vi "Init AC Source.vi"(6 "General Settings:Timeout Value":u32=2000, 8 "error in (no error)":errorcluster, 9 "AC sync source":T1, 11 "AC source":T1) -> (0 "error out":errorcluster, 1 "AC sync source out":T1, 2 "Init status":string, 3 "AC source out":T1)   [LabVIEW 2020]
doc: "Initialize the driver of the selected AC source."
uses:
  Type definitions/AC Source.ctl
  Type definitions/AC Source type.ctl
  external libraries/Fluke 5XXX Series Multicalibrator/Fluke 5XXX Series Multicalibrators.lvlib
  external libraries/AWG/AFG3000/Tektronix AFG 3000 Series.lvlib
  external libraries/AWG/Agilent 33XXX Series/Agilent 33XXX Series.lvlib
  external libraries/AWG/Agilent 3352X Series/Agilent 3352X Series.lvlib
panel:
  in  "General Settings:Timeout Value 2":u32=2000
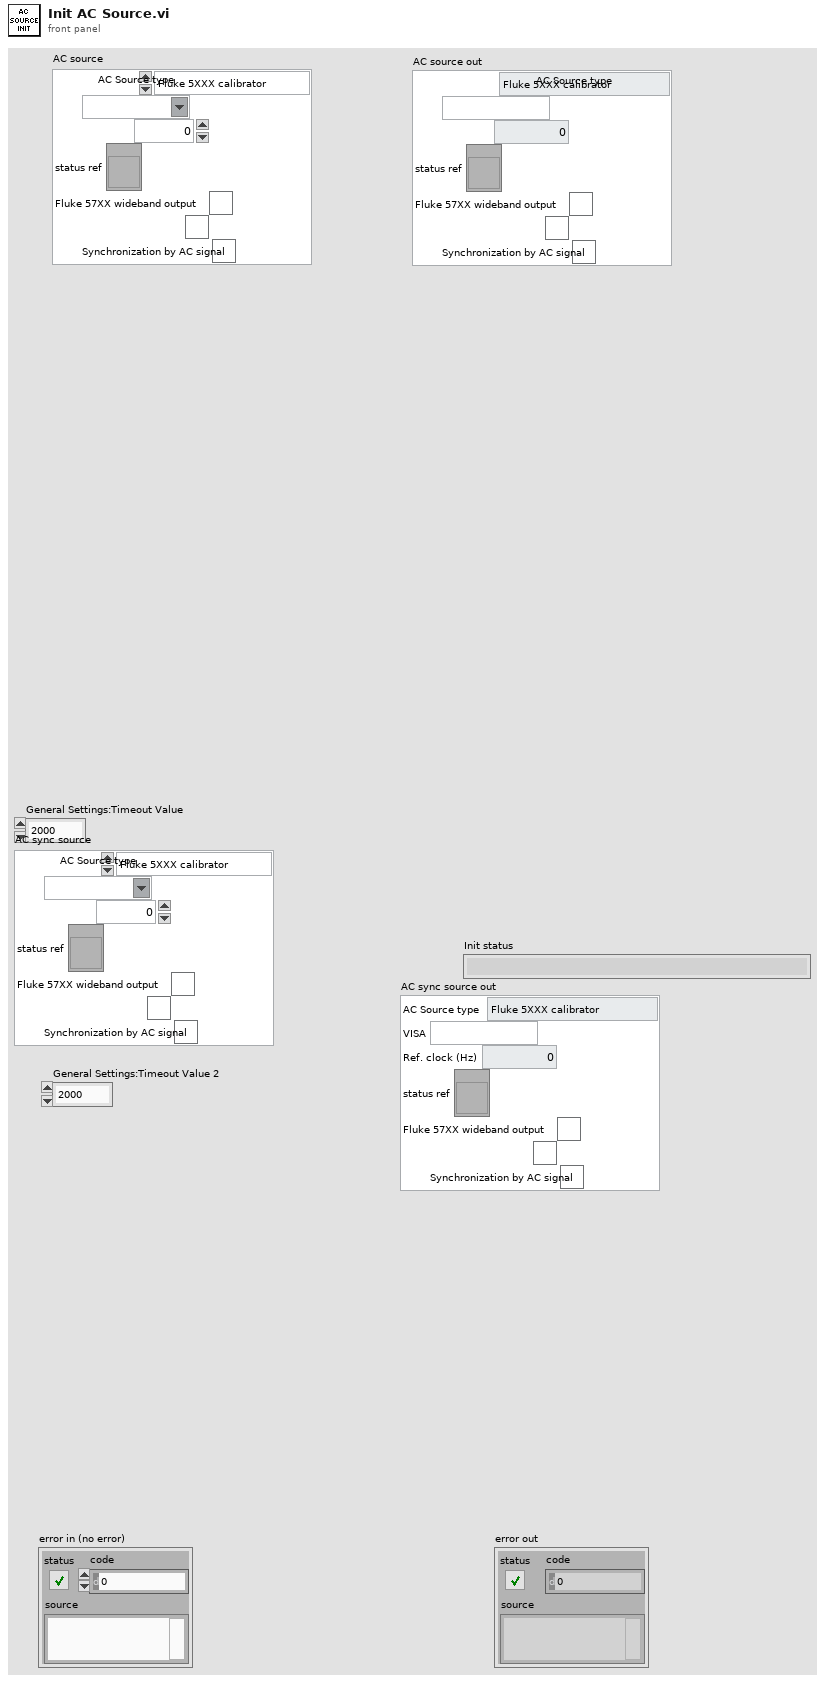
[diagram p1: front panel]
types:
  T1 = typedef "AC Source.ctl" = cluster{"AC Source type":T2, "VISA":refnum<visa-resource-name>, "Ref. clock (Hz)":dbl, "status ref":refnum<vi>, "Fluke 57XX wideband output":bool, "Fluke 57XX ignore errors":bool, "Synchronization by AC signal":bool}
  T2 = typedef "AC Source type.ctl" = enum16{"Fluke 5XXX calibrator", "Tektronix AFG3000 series", "dummy", "Agilent 331xxA to 332xxA", "Agilent 335xxA to 336xxA"}
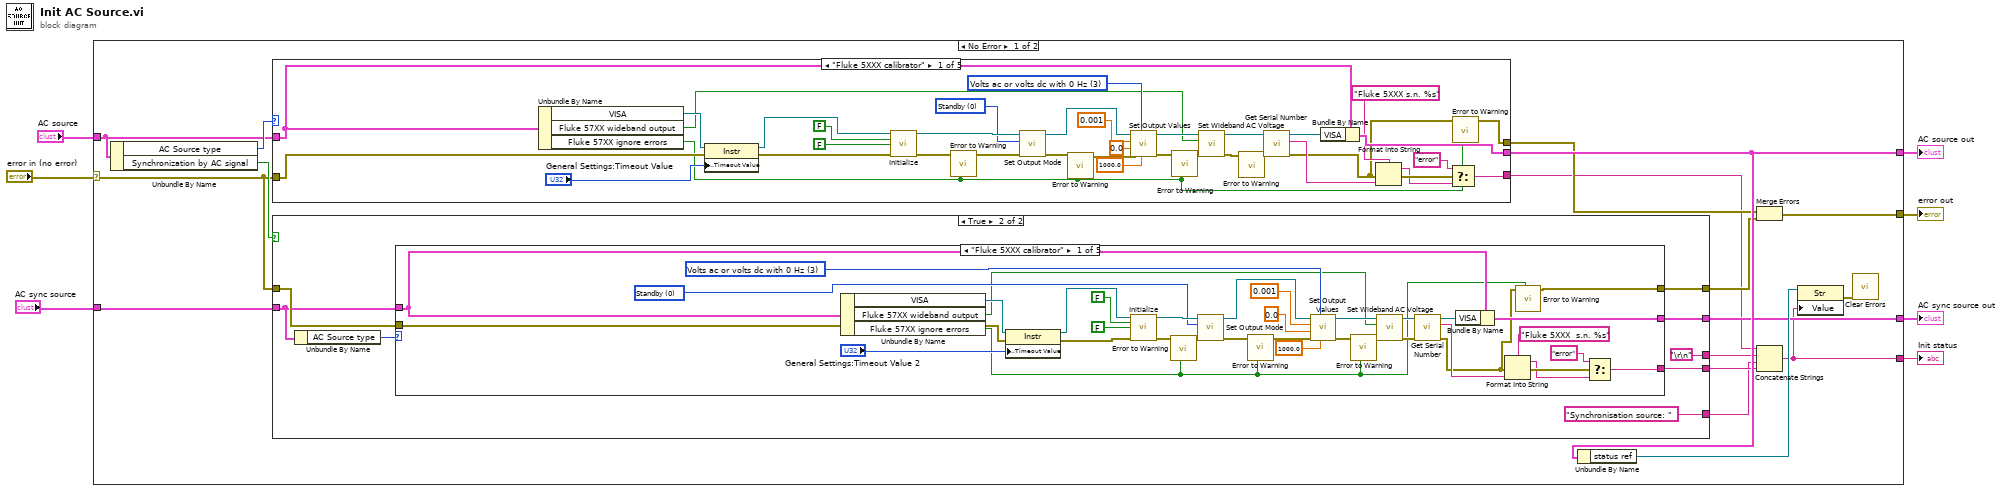
[diagram p0: block diagram]
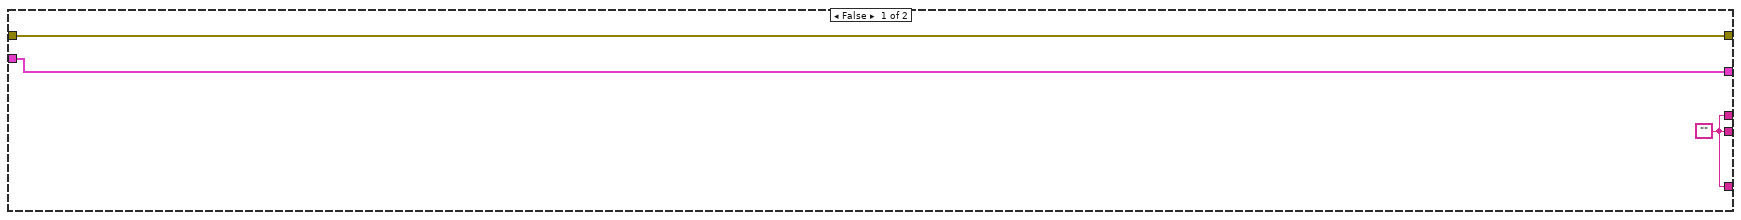
[diagram p2: hidden frame]
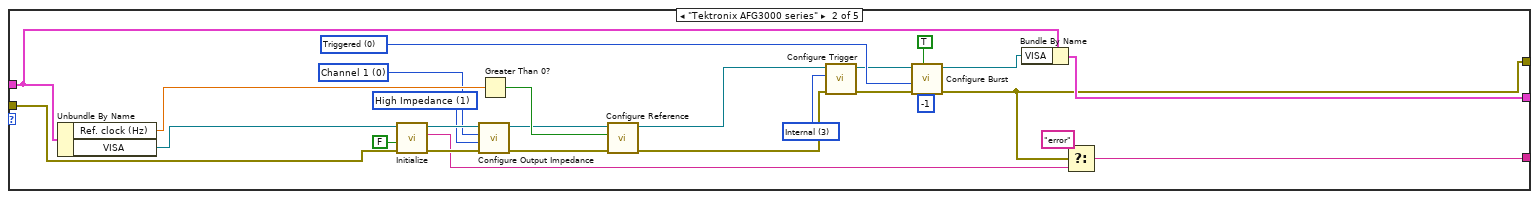
[diagram p3: hidden frame]
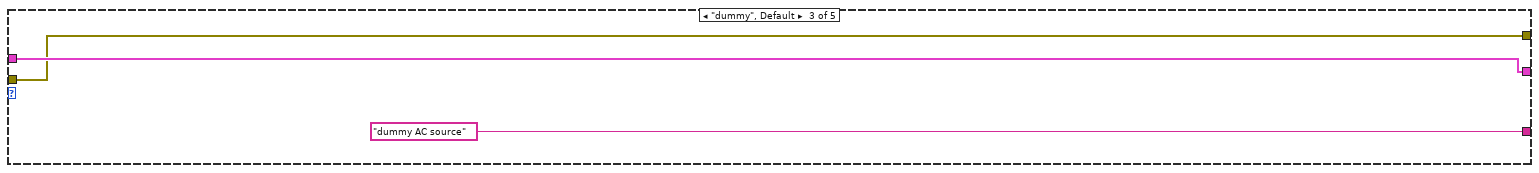
[diagram p4: hidden frame]
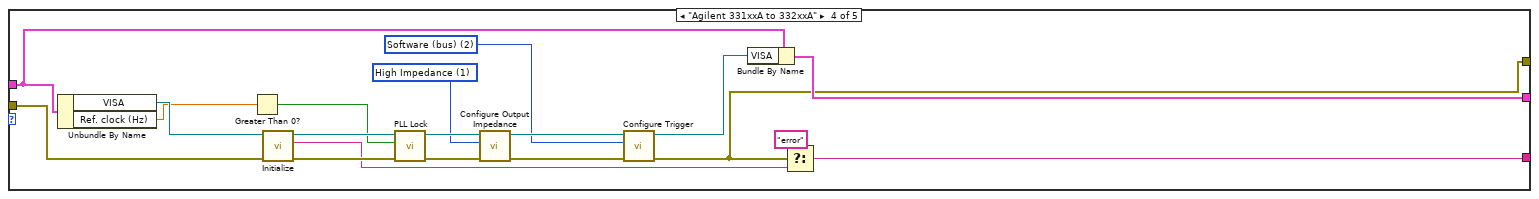
[diagram p5: hidden frame]
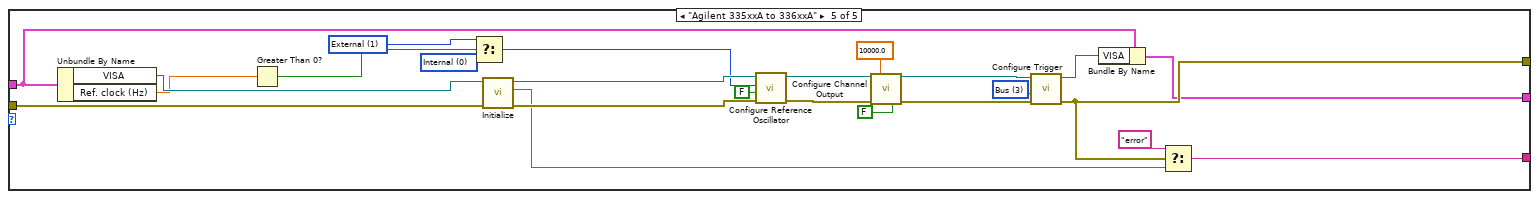
[diagram p6: hidden frame]
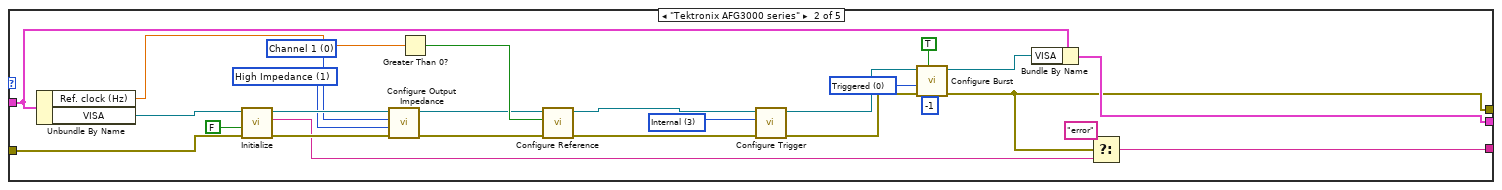
[diagram p7: hidden frame]
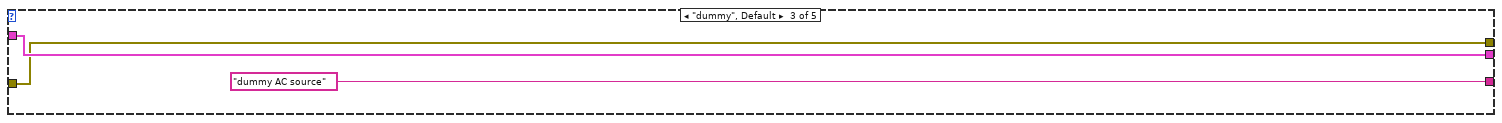
[diagram p8: hidden frame]
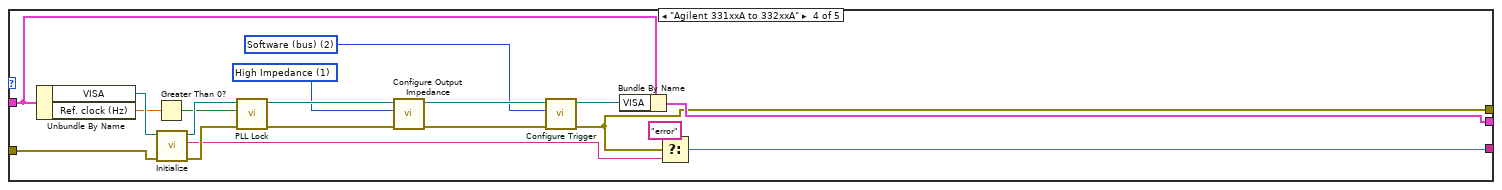
[diagram p9: hidden frame]
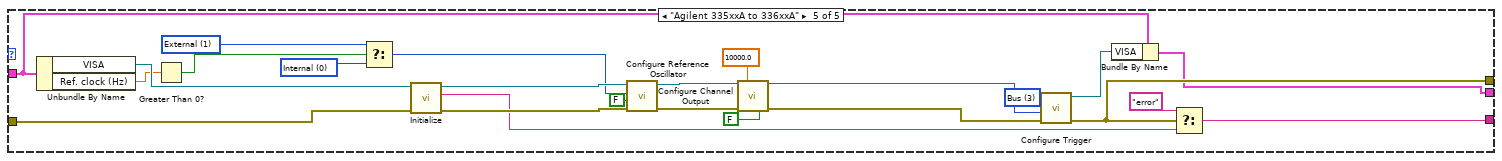
[diagram p10: hidden frame]
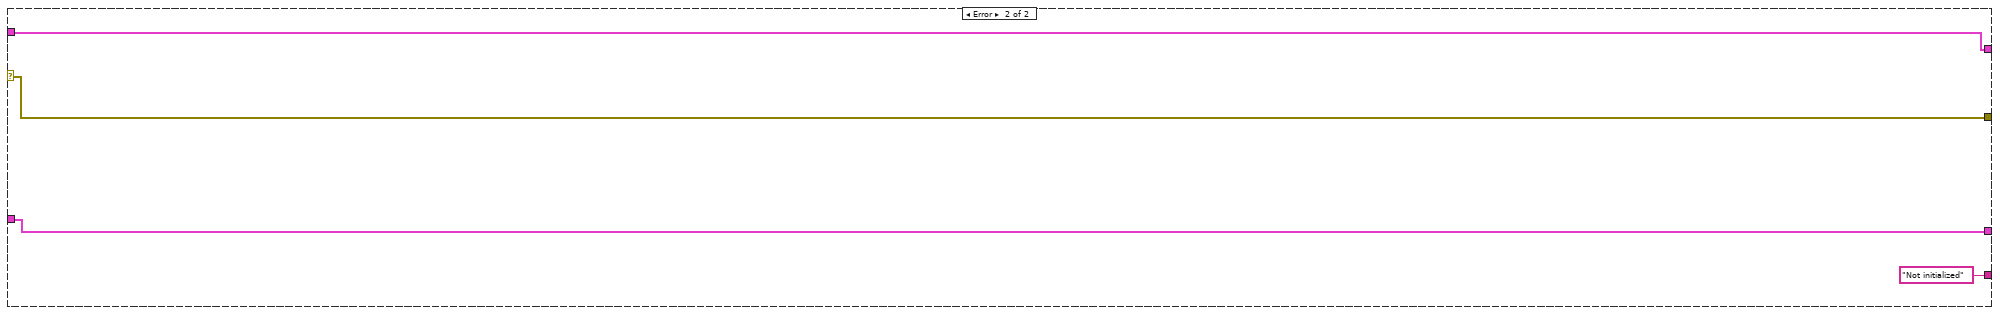
[diagram p11: hidden frame]
diagram:
  n1 = case shown="No Error" "error in (no error)" {
    selector: "error in (no error)" -> [w17 w255]
    tunnel: [w13 w255] -> w7
    tunnel: "AC source" -> [w23 w256]
    tunnel: [w22 w256] -> w5
    tunnel: [w11 "Not initialized" ("idn string")] -> w4
    tunnel: "AC sync source" -> [w18 w253]
    tunnel: [w16 w253] -> w1
    frame No Error {
      n2 = Unbundle By Name(w23) -> ("AC Source type"=w24:T2, "Synchronization by AC signal"=w19:bool)
      n3 = case shown="\"Fluke 5XXX calibrator\"" w24 {
        tunnel: w17 -> [w163 w200 w208 w220 w235]
        tunnel: [w145 w183 w208 w212 w233] -> w15
        tunnel: w23 -> [w180 w186 w209 w215 w230]
        tunnel: [w179 w185 w209 w214 w229] -> w22
        tunnel: [w171 w182 "dummy AC source" ("idn string") w210 w232] -> w12
        frame "Fluke 5XXX calibrator" {
          w174 = u32 3 items=["Amplitude", "Volts dc or update volts ac", "Volts ac dBm update", "Volts ac or volts dc with 0 Hz", "Volts ac in dBm", "Current dc or update current ac", "Current ac", "Update frequency", "Resistance", "Capacitance", "Temperature (Celsius)", "Temperature (Fahrenheit)", "Power dc or update power ac", "Power ac", "Dual volts dc or update dual ac", "Dual volts ac in volts", "Power ac in dBm update", "Power ac in dBm", "Dual volts ac in dBm update", "Dual volts ac in dBm"] ("Output Value(s) (0 - Amplitude)")
          w175 = u32 0 items=["Standby", "Operate"] ("Output Mode (0: Standby)")
          n4 = Unbundle By Name(w180) -> ("VISA"=w161:refnum<visa-resource-name>, "Fluke 57XX wideband output"=w157:bool, "Fluke 57XX ignore errors"=w146:bool)
          n5 = property class="Instr"(reference=w161, error in=w163, "General Settings:Timeout Value"="General Settings:Timeout Value") -> (reference out=w160:refnum<visa-resource-name>, error out=w162:errorcluster)
          n6 = call "Initialize.vi"("VISA resource name"=w160, "ID Query (T: Check)"=FALSE, "Reset (T: Reset)"=FALSE, "error in (no error)"=w162) -> ("VISA resource name out"=w177:refnum<visa-resource-name>, "error out"=w154:errorcluster)  [unwired: 10 in]
          n7 = call "Error to Warning.vi"("Change to warning?"=w146, "error in (no error)"=w154) -> ("error out"=w153:errorcluster)  [unwired: 9 in]
          n8 = call "Set Output Mode.vi"("error in (no error)"=w153, "Output Mode (0: Standby)"=w175, "VISA resource name"=w177) -> ("error out"=w152:errorcluster, "VISA resource name out"=w176:refnum<visa-resource-name>)  [unwired: 7 in]
          n9 = call "Error to Warning.vi"("Change to warning?"=w146, "error in (no error)"=w152) -> ("error out"=w151:errorcluster)  [unwired: 9 in]
          n10 = call "Set Output Values.vi"("Fundamental Frequency (0.0 Hz)"=1000.0, "Output Value(s) (0 - Amplitude)"=w174, "error in (no error)"=w151, "Secondary Value (0.0)"=0.0, "Primary Value (0.0)"=0.001, "VISA resource name"=w176) -> ("error out"=w150:errorcluster, "VISA resource name out"=w158:refnum<visa-resource-name>)  [unwired: 4 in]
          n11 = call "Error to Warning.vi"("Change to warning?"=w146, "error in (no error)"=w150) -> ("error out"=w149:errorcluster)  [unwired: 9 in]
          n12 = call "Set Wideband AC Voltage.vi"("error in (no error)"=w149, "Wideband Mode (F: Off)"=w157, "VISA resource name"=w158) -> ("error out"=w148:errorcluster, "VISA resource name out"=w159:refnum<visa-resource-name>)  [unwired: 7 in]
          n13 = call "Error to Warning.vi"("error in (no error)"=w148) -> ("error out"=w147:errorcluster)  [unwired: 10 in]
          n14 = call "Get Serial Number.vi"("error in (no error)"=w147, "VISA resource name"=w159) -> ("error out"=w144:errorcluster, "Serial Number"=w168:string, "VISA resource name out"=w170:refnum<visa-resource-name>)  [unwired: 7 in]
          n15 = Bundle By Name(cluster=w180, "VISA"=w170) -> (w179:T1)
          n16 = Format Into String(format string="Fluke 5XXX s.n. %s", error in=w144, w168) -> (resulting string=w166:string, error out=w167:errorcluster)  [unwired: 1 in]
          n17 = Select(t="error" ("idn string"), s=w167, f=w166) -> (s? t:f=w171:string)
          n18 = call "Error to Warning.vi"("Change to warning?"=w146, "error in (no error)"=w144) -> ("error out"=w145:errorcluster)  [unwired: 9 in]
        }
        frame "Tektronix AFG3000 series" {
          w192 = u16 1 items=["50 Ohm", "High Impedance", "Customized"] ("Impedance (0: 50 Ohm)")
          w193 = u16 0 items=["Channel 1", "Channel2"] ("Channel (0: Channel 1)")
          w201 = u16 3 items=["Internal"=3, "External"=1] ("Trigger Source (3:Internal)")
          w206 = u16 0 items=["Triggered", "Gated"] ("Burst Mode (0: Triggered)")
          n19 = Unbundle By Name(w186) -> ("Ref. clock (Hz)"=w197:dbl, "VISA"=w199:refnum<visa-resource-name>)
          n20 = call "Initialize.vi"("error in (no error)"=w200, "Reset (True)"=FALSE, "VISA resource name"=w199) -> ("error out"=w195:errorcluster, "idn string"=w181:string, "VISA resource name out"=w194:refnum<visa-resource-name>)  [unwired: 6 in]
          n21 = call "Configure Output Impedance.vi"("error in (no error)"=w195, "Impedance (0: 50 Ohm)"=w192, "Channel (0: Channel 1)"=w193, "VISA resource name"=w194) -> ("error out"=w191:errorcluster, "VISA resource name out"=w190:refnum<visa-resource-name>)  [unwired: 6 in]
          n22 = Greater Than 0?(x=w197) -> (x > 0?=w196:bool)
          n23 = call "Configure Reference.vi"("error in (no error)"=w191, "external clock"=w196, "VISA resource name"=w190) -> ("error out"=w188:errorcluster, "VISA resource name out"=w189:refnum<visa-resource-name>)  [unwired: 7 in]
          n24 = call "Configure Trigger.vi"("error in (no error)"=w188, "Trigger Source (3:Internal)"=w201, "VISA resource name"=w189) -> ("error out"=w203:errorcluster, "VISA resource name out"=w202:refnum<visa-resource-name>)  [unwired: 7 in]
          n25 = call "Configure Burst.vi"("Burst Count (5)"=-1, "Enable Burst (T: Enable)"=TRUE, "error in (no error)"=w203, "Burst Mode (0: Triggered)"=w206, "VISA resource name"=w202) -> ("error out"=w183:errorcluster, "VISA resource name out"=w187:refnum<visa-resource-name>)  [unwired: 5 in]
          n26 = Bundle By Name(cluster=w186, "VISA"=w187) -> (w185:T1)
          n27 = Select(t="error" ("idn string"), s=w183, f=w181) -> (s? t:f=w182:string)
        }
        frame "dummy", Default {
        }
        frame "Agilent 331xxA to 332xxA" {
          w221 = u16 2 items=["Internal", "External", "Software (bus)"] ("Trigger Source (0: Internal)")
          w224 = u16 1 items=["50 Ohms", "High Impedance", "User Defined"] ("Impedance (0: 50 Ohms)")
          n28 = Unbundle By Name(w215) -> ("VISA"=w219:refnum<visa-resource-name>, "Ref. clock (Hz)"=w218:dbl)
          n29 = Greater Than 0?(x=w218) -> (x > 0?=w217:bool)
          n30 = call "Initialize.vi"("error in (no error)"=w220, "VISA resource name"=w219) -> ("error out"=w228:errorcluster, "idn string"=w211:string, "VISA resource name out"=w227:refnum<visa-resource-name>)  [unwired: 7 in]
          n31 = call "PLL Lock.vi"("error in (no error)"=w228, "PLL lock  (T: Enable)"=w217, "VISA resource name"=w227) -> ("error out"=w226:errorcluster, "VISA resource name out"=w225:refnum<visa-resource-name>)  [unwired: 7 in]
          n32 = call "Configure Output Impedance.vi"("error in (no error)"=w226, "Impedance (0: 50 Ohms)"=w224, "VISA resource name"=w225) -> ("error out"=w223:errorcluster, "VISA resource name out"=w222:refnum<visa-resource-name>)  [unwired: 7 in]
          n33 = call "Configure Trigger.vi"("error in (no error)"=w223, "Trigger Source (0: Internal)"=w221, "VISA resource name"=w222) -> ("error out"=w212:errorcluster, "VISA resource name out"=w216:refnum<visa-resource-name>)  [unwired: 7 in]
          n34 = Bundle By Name(cluster=w215, "VISA"=w216) -> (w214:T1)
          n35 = Select(t="error" ("idn string"), s=w212, f=w211) -> (s? t:f=w210:string)
        }
        frame "Agilent 335xxA to 336xxA" {
          w238 = 3 items=["Immediate", "External", "Timer", "Bus"] ("Trigger Source (0: Immediate)")
          w243 = 1 items=["Internal", "External"] ("Source (0: Internal)")
          w242 = 0 items=["Internal", "External"] ("Source (0: Internal)")
          n36 = Unbundle By Name(w230) -> ("VISA"=w252:refnum<visa-resource-name>, "Ref. clock (Hz)"=w237:dbl)
          n37 = Greater Than 0?(x=w237) -> (x > 0?=w236:bool)
          n38 = Select(t=w243, s=w236, f=w242) -> (s? t:f=w244:i32)
          n39 = call "Initialize.vi"("error in (no error)"=w235, "VISA resource name"=w252) -> ("error out"=w250:errorcluster, "idn string"=w231:string, "VISA resource name out"=w251:refnum<visa-resource-name>)  [unwired: 7 in]
          n40 = call "Configure Reference Oscillator.vi"("error in (no error)"=w250, "Source Auto Selection(T: Enable)"=FALSE, "Source (0: Internal)"=w244, "VISA resource name"=w251) -> ("error out"=w249:errorcluster, "VISA resource name out"=w248:refnum<visa-resource-name>)  [unwired: 6 in]
          n41 = call "Configure Channel Output.vi"("VISA resource name"=w248, "Output Impedance (50 Ohm)"=10000.0, "error in (no error)"=w249, "Enable Voltage Limit (T: Enable)"=FALSE) -> ("VISA resource name out"=w241:refnum<visa-resource-name>, "error out"=w239:errorcluster)  [unwired: 10 in]
          n42 = call "Configure Trigger.vi"("error in (no error)"=w239, "Trigger Source (0: Immediate)"=w238, "VISA resource name"=w241) -> ("error out"=w233:errorcluster, "VISA resource name out"=w240:refnum<visa-resource-name>)  [unwired: 7 in]
          n43 = Bundle By Name(cluster=w230, "VISA"=w240) -> (w229:T1)
          n44 = Select(t="error" ("idn string"), s=w233, f=w231) -> (s? t:f=w232:string)
        }
      }
      n45 = case shown="True" w19 {
        tunnel: w18 -> [w26 w29]
        tunnel: w17 -> [w27 w35]
        tunnel: [w27 w34] -> w14
        tunnel: [w26 w33] -> w16
        tunnel: [w25 w32] -> w10
        tunnel: [w25 "Synchronisation source: " ("string")] -> w9
        tunnel: [w25 "\r\n"] -> w8
        frame False {
          w25 = ""
        }
        frame True {
          n46 = Unbundle By Name(w29) -> ("AC Source type"=w28:T2)
          n47 = case shown="\"Fluke 5XXX calibrator\"" w28 {
            tunnel: w35 -> [w53 w91 w99 w111 w126]
            tunnel: [w39 w74 w99 w103 w124] -> w34
            tunnel: w29 -> [w71 w77 w100 w106 w121]
            tunnel: [w70 w76 w100 w105 w120] -> w33
            tunnel: [w61 w73 "dummy AC source" ("idn string") w101 w123] -> w32
            frame "Fluke 5XXX calibrator" {
              w65 = u32 3 items=["Amplitude", "Volts dc or update volts ac", "Volts ac dBm update", "Volts ac or volts dc with 0 Hz", "Volts ac in dBm", "Current dc or update current ac", "Current ac", "Update frequency", "Resistance", "Capacitance", "Temperature (Celsius)", "Temperature (Fahrenheit)", "Power dc or update power ac", "Power ac", "Dual volts dc or update dual ac", "Dual volts ac in volts", "Power ac in dBm update", "Power ac in dBm", "Dual volts ac in dBm update", "Dual volts ac in dBm"] ("Output Value(s) (0 - Amplitude)")
              w66 = u32 0 items=["Standby", "Operate"] ("Output Mode (0: Standby)")
              n48 = Unbundle By Name(w71) -> ("VISA"=w51:refnum<visa-resource-name>, "Fluke 57XX wideband output"=w46:bool, "Fluke 57XX ignore errors"=w37:bool)
              n49 = property class="Instr"(reference=w51, error in=w53, "General Settings:Timeout Value"="General Settings:Timeout Value 2") -> (reference out=w50:refnum<visa-resource-name>, error out=w52:errorcluster)
              n50 = call "Initialize.vi"("VISA resource name"=w50, "ID Query (T: Check)"=FALSE, "Reset (T: Reset)"=FALSE, "error in (no error)"=w52) -> ("VISA resource name out"=w68:refnum<visa-resource-name>, "error out"=w45:errorcluster)  [unwired: 10 in]
              n51 = call "Error to Warning.vi"("Change to warning?"=w37, "error in (no error)"=w45) -> ("error out"=w43:errorcluster)  [unwired: 9 in]
              n52 = call "Set Output Mode.vi"("error in (no error)"=w43, "Output Mode (0: Standby)"=w66, "VISA resource name"=w68) -> ("error out"=w42:errorcluster, "VISA resource name out"=w67:refnum<visa-resource-name>)  [unwired: 7 in]
              n53 = call "Error to Warning.vi"("Change to warning?"=w37, "error in (no error)"=w42) -> ("error out"=w41:errorcluster)  [unwired: 9 in]
              n54 = call "Set Output Values.vi"("Fundamental Frequency (0.0 Hz)"=1000.0, "Output Value(s) (0 - Amplitude)"=w65, "error in (no error)"=w41, "Secondary Value (0.0)"=0.0, "Primary Value (0.0)"=0.001, "VISA resource name"=w67) -> ("error out"=w44:errorcluster, "VISA resource name out"=w47:refnum<visa-resource-name>)  [unwired: 4 in]
              n55 = call "Error to Warning.vi"("Change to warning?"=w37, "error in (no error)"=w44) -> ("error out"=w40:errorcluster)  [unwired: 9 in]
              n56 = call "Set Wideband AC Voltage.vi"("error in (no error)"=w40, "Wideband Mode (F: Off)"=w46, "VISA resource name"=w47) -> ("error out"=w49:errorcluster, "VISA resource name out"=w48:refnum<visa-resource-name>)  [unwired: 7 in]
              n57 = call "Get Serial Number.vi"("error in (no error)"=w49, "VISA resource name"=w48) -> ("error out"=w38:errorcluster, "Serial Number"=w58:string, "VISA resource name out"=w60:refnum<visa-resource-name>)  [unwired: 7 in]
              n58 = Bundle By Name(cluster=w71, "VISA"=w60) -> (w70:T1)
              n59 = Format Into String(format string="Fluke 5XXX  s.n. %s", error in=w38, w58) -> (resulting string=w56:string, error out=w57:errorcluster)  [unwired: 1 in]
              n60 = call "Error to Warning.vi"("Change to warning?"=w37, "error in (no error)"=w38) -> ("error out"=w39:errorcluster)  [unwired: 9 in]
              n61 = Select(t="error" ("idn string"), s=w57, f=w56) -> (s? t:f=w61:string)
            }
            frame "Tektronix AFG3000 series" {
              w83 = u16 1 items=["50 Ohm", "High Impedance", "Customized"] ("Impedance (0: 50 Ohm)")
              w84 = u16 0 items=["Channel 1", "Channel2"] ("Channel (0: Channel 1)")
              w92 = u16 3 items=["Internal"=3, "External"=1] ("Trigger Source (3:Internal)")
              w97 = u16 0 items=["Triggered", "Gated"] ("Burst Mode (0: Triggered)")
              n62 = Unbundle By Name(w77) -> ("Ref. clock (Hz)"=w88:dbl, "VISA"=w90:refnum<visa-resource-name>)
              n63 = call "Initialize.vi"("error in (no error)"=w91, "Reset (True)"=FALSE, "VISA resource name"=w90) -> ("error out"=w86:errorcluster, "idn string"=w72:string, "VISA resource name out"=w85:refnum<visa-resource-name>)  [unwired: 6 in]
              n64 = call "Configure Output Impedance.vi"("error in (no error)"=w86, "Impedance (0: 50 Ohm)"=w83, "Channel (0: Channel 1)"=w84, "VISA resource name"=w85) -> ("error out"=w82:errorcluster, "VISA resource name out"=w81:refnum<visa-resource-name>)  [unwired: 6 in]
              n65 = Greater Than 0?(x=w88) -> (x > 0?=w87:bool)
              n66 = call "Configure Reference.vi"("error in (no error)"=w82, "external clock"=w87, "VISA resource name"=w81) -> ("error out"=w79:errorcluster, "VISA resource name out"=w80:refnum<visa-resource-name>)  [unwired: 7 in]
              n67 = call "Configure Trigger.vi"("error in (no error)"=w79, "Trigger Source (3:Internal)"=w92, "VISA resource name"=w80) -> ("error out"=w94:errorcluster, "VISA resource name out"=w93:refnum<visa-resource-name>)  [unwired: 7 in]
              n68 = call "Configure Burst.vi"("Burst Count (5)"=-1, "Enable Burst (T: Enable)"=TRUE, "error in (no error)"=w94, "Burst Mode (0: Triggered)"=w97, "VISA resource name"=w93) -> ("error out"=w74:errorcluster, "VISA resource name out"=w78:refnum<visa-resource-name>)  [unwired: 5 in]
              n69 = Bundle By Name(cluster=w77, "VISA"=w78) -> (w76:T1)
              n70 = Select(t="error" ("idn string"), s=w74, f=w72) -> (s? t:f=w73:string)
            }
            frame "dummy", Default {
            }
            frame "Agilent 331xxA to 332xxA" {
              w112 = u16 2 items=["Internal", "External", "Software (bus)"] ("Trigger Source (0: Internal)")
              w115 = u16 1 items=["50 Ohms", "High Impedance", "User Defined"] ("Impedance (0: 50 Ohms)")
              n71 = Unbundle By Name(w106) -> ("VISA"=w110:refnum<visa-resource-name>, "Ref. clock (Hz)"=w109:dbl)
              n72 = Greater Than 0?(x=w109) -> (x > 0?=w108:bool)
              n73 = call "Initialize.vi"("error in (no error)"=w111, "VISA resource name"=w110) -> ("error out"=w119:errorcluster, "idn string"=w102:string, "VISA resource name out"=w118:refnum<visa-resource-name>)  [unwired: 7 in]
              n74 = call "PLL Lock.vi"("error in (no error)"=w119, "PLL lock  (T: Enable)"=w108, "VISA resource name"=w118) -> ("error out"=w117:errorcluster, "VISA resource name out"=w116:refnum<visa-resource-name>)  [unwired: 7 in]
              n75 = call "Configure Output Impedance.vi"("error in (no error)"=w117, "Impedance (0: 50 Ohms)"=w115, "VISA resource name"=w116) -> ("error out"=w114:errorcluster, "VISA resource name out"=w113:refnum<visa-resource-name>)  [unwired: 7 in]
              n76 = call "Configure Trigger.vi"("error in (no error)"=w114, "Trigger Source (0: Internal)"=w112, "VISA resource name"=w113) -> ("error out"=w103:errorcluster, "VISA resource name out"=w107:refnum<visa-resource-name>)  [unwired: 7 in]
              n77 = Bundle By Name(cluster=w106, "VISA"=w107) -> (w105:T1)
              n78 = Select(t="error" ("idn string"), s=w103, f=w102) -> (s? t:f=w101:string)
            }
            frame "Agilent 335xxA to 336xxA" {
              w129 = 3 items=["Immediate", "External", "Timer", "Bus"] ("Trigger Source (0: Immediate)")
              w134 = 1 items=["Internal", "External"] ("Source (0: Internal)")
              w133 = 0 items=["Internal", "External"] ("Source (0: Internal)")
              n79 = Unbundle By Name(w121) -> ("VISA"=w143:refnum<visa-resource-name>, "Ref. clock (Hz)"=w128:dbl)
              n80 = Greater Than 0?(x=w128) -> (x > 0?=w127:bool)
              n81 = Select(t=w134, s=w127, f=w133) -> (s? t:f=w135:i32)
              n82 = call "Initialize.vi"("error in (no error)"=w126, "VISA resource name"=w143) -> ("error out"=w141:errorcluster, "idn string"=w122:string, "VISA resource name out"=w142:refnum<visa-resource-name>)  [unwired: 7 in]
              n83 = call "Configure Reference Oscillator.vi"("error in (no error)"=w141, "Source Auto Selection(T: Enable)"=FALSE, "Source (0: Internal)"=w135, "VISA resource name"=w142) -> ("error out"=w140:errorcluster, "VISA resource name out"=w139:refnum<visa-resource-name>)  [unwired: 6 in]
              n84 = call "Configure Channel Output.vi"("VISA resource name"=w139, "Output Impedance (50 Ohm)"=10000.0, "error in (no error)"=w140, "Enable Voltage Limit (T: Enable)"=FALSE) -> ("VISA resource name out"=w132:refnum<visa-resource-name>, "error out"=w130:errorcluster)  [unwired: 10 in]
              n85 = call "Configure Trigger.vi"("error in (no error)"=w130, "Trigger Source (0: Immediate)"=w129, "VISA resource name"=w132) -> ("error out"=w124:errorcluster, "VISA resource name out"=w131:refnum<visa-resource-name>)  [unwired: 7 in]
              n86 = Bundle By Name(cluster=w121, "VISA"=w131) -> (w120:T1)
              n87 = Select(t="error" ("idn string"), s=w124, f=w122) -> (s? t:f=w123:string)
            }
          }
        }
      }
      n88 = Unbundle By Name(w22) -> ("status ref"=w21:refnum<vi>)
      n89 = Merge Errors(w15, w14) -> (w13:errorcluster)
      n90 = Concatenate Strings(w12, w8, w9, w10) -> (w11:string)
      n91 = property class="Str"(reference=w21, "Value"=w11) -> (error out=w20:errorcluster)  [unwired: 1 in, 1 out]
      n92 = call <vilib>:"Clear Errors.vi"("error in (no error)"=w20) -> ()  [unwired: 5 in, 2 out]
    }
    frame Error {
    }
  }
  "error out" <- w7
  "AC source out" <- w5
  "Init status" <- w4
  "AC sync source out" <- w1
